vi "CSM - Sync with File.vi"(7 "error in (no error)":errorcluster) -> (1 "error out":errorcluster)   [LabVIEW 2017, in "INI-Static-Variable-Support.lvlib"]
uses:
  INI-Static-Variable-Support.lvlib
  _Support/_fgv-oper.ctl
  _Support/global-csm-ini-db-change-flag.vi
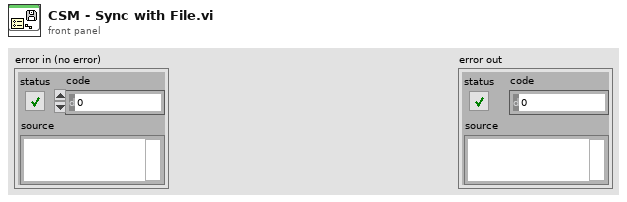
[diagram p1: front panel]
types:
  T1 = typedef "_fgv-oper.ctl" = enum16{"Read", "Write", "Sync"}
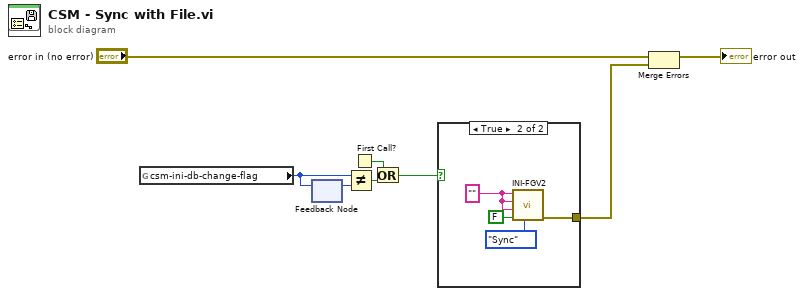
[diagram p0: block diagram]
diagram:
  n1 = global read "global-csm-ini-db-change-flag.vi" "csm-ini-db-change-flag"() -> (w6:u32)
  n2 = feedback #1() -> (w5:u32)  [unwired: 1 in]
  n3 = feedback-in #1(w6) -> ()
  n4 = Not Equal?(x=w6, y=w5) -> (x != y?=w4:bool)
  n5 = First Call?() -> (First Call?: T/F=w3:bool)
  n6 = Or(x=w3, y=w4) -> (x .or. y?=w2:bool)
  n7 = case shown="True" w2 {
    tunnel: [_ w9] -> w1
    frame False {
    }
    frame True {
      w12 = "" (">> Variable Name >>")
      n8 = call "INI-FGV2.vi"("Enum"=_fgv-oper."Sync", "Raw String? (F)"=FALSE, ">> Section >>"=w12, ">> Default Value >>"=w12, ">> Variable Name >>"=w12) -> ("error out"=w9:errorcluster)  [unwired: 4 in, 2 out]
    }
  }
  n9 = Merge Errors("error in (no error)", w1) -> (→"error out":errorcluster)
